vi "Post-Process.vi"(11 "Arilou in":refnum<class "Arilou.lvclass">) -> (2 "New Elements":refnum<class "Element.lvclass">[](array[class]), 3 "Arilou out":refnum<class "Arilou.lvclass">)   [LabVIEW 2021, in "Arilou.lvclass"]
uses:
  Arilou.lvclass
  Element/Element.lvclass
  Ship/Ship.lvclass
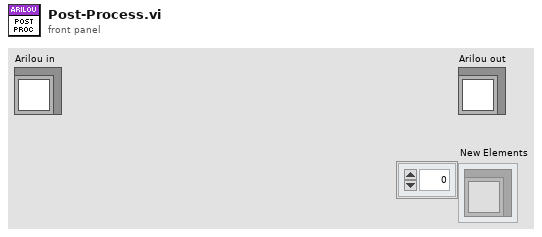
[diagram p1: front panel]
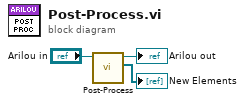
[diagram p0: block diagram]
diagram:
  n1 = call-parent "Post-Process.vi"("Ship in"="Arilou in") -> ("New Elements"=→"New Elements":refnum<class "Element.lvclass">[], "Ship out"=→"Arilou out":refnum<class "Arilou.lvclass">)  [unwired: 9 in]
